vi "Teardown_Tests.vi"(8 "error in":errorcluster, 10 "Module Was Already Running?":bool, 11 "horiba.lvlib:GenericDevice":refnum<class "GenericDevice.lvclass">) -> (0 "error out":errorcluster, 2 "device is open?":bool)   [LabVIEW 2023, in "horiba.test.lvlib"]
uses:
  Classes/GenericDevice/GenericDevice.lvclass
  horiba.test.lvlib
  Classes/DeviceManager/DeviceManager.lvlib
panel:
  # "Connector Pane"
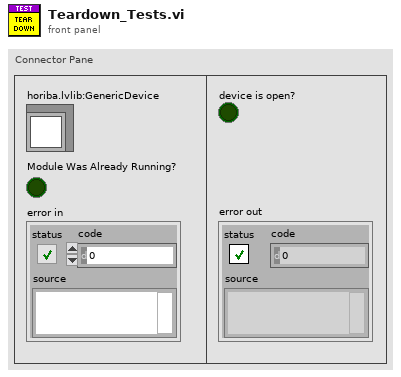
[diagram p1: front panel]
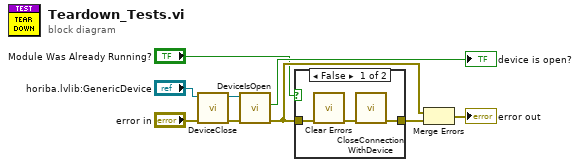
[diagram p0: block diagram]
diagram:
  n1 = call-dynamic "DeviceClose.vi"("error in (no error)"="error in", "GenericDevice in"="horiba.lvlib:GenericDevice") -> ("error out"=w7:errorcluster, "GenericDevice out"=w8:refnum<class "GenericDevice.lvclass">)  [unwired: 5 in, 3 out]
  n2 = call-dynamic "DeviceIsOpen.vi"("error in (no error)"=w7, "GenericDevice in"=w8) -> ("error out"=w4:errorcluster, "device is open?"=→"device is open?":bool)  [unwired: 6 in, 2 out]
  n3 = case shown="False" "Module Was Already Running?" {
    tunnel: w4 -> [w11 w13]
    tunnel: [w10 w13] -> w2
    frame False {
      n4 = call <vilib>:"Clear Errors.vi"("error in (no error)"=w11) -> ("error out"=w12:errorcluster)  [unwired: 5 in, 1 out]
      n5 = call "CloseConnectionWithDevice.vi"("error in (no error)"=w12) -> ("error out"=w10:errorcluster)  [unwired: 10 in]
    }
    frame True {
    }
  }
  n6 = Merge Errors(w4, w2) -> (→"error out":errorcluster)
